vi "AR-Axis-update-parameters-GUI.vi"(8 "error in":errorcluster, 11 "Com":refnum<visa-resource-name>) -> (0 "error out":errorcluster, 1 "Axis":string[](array[string]), 2 "Connected Devices":string[](array[string]), 3 "Device Info":T4(array[cluster]) {"Microstep Size" format="%#_6f"})   [LabVIEW 2021]
uses:
  Automation/Zaber Stage/Controls/Zaber-basic-settings.ctl
  Automation/Zaber Stage/Controls/Zaber-all-settings.ctl
  <instrlib>/Zaber A Series/Public/Utility/Low Level/Convert Device Units to Position Units.vi
  <instrlib>/Zaber A Series/Public/Utility/Low Level/Convert Device Units to Speed Units.vi
  <instrlib>/Zaber A Series/Public/Utility/Low Level/Convert Device Units to Acceleration.vi
  <instrlib>/Zaber A Series/Zaber A Series.lvlib
panel:
  in  "Axis":string(combo)
  in  "All Settings":T1="cloop.duration.max"
  in  "Basic Settings":T2="comm.checksum"
  in  "Physical Units":T3(ring)
  out "To Physical Units":string
  in  "From Device":i32
  out "To Device Units":string
  in  "From Physical":dbl
  in  "Convert":enum16{"Position", "Speed", "Acceleration"}(ring)
  in  "Quit":bool
  out "Action":string
  in  "Set":bool
  in  "Get":bool
  out "Setting readback":string
  in  "Cmd parameters":string
  in  "Setting cmd":string(combo)
  in  "All/Basic(T)":bool=TRUE
  in  "Device#":string(combo)
  out "Settings":string[](array[string])
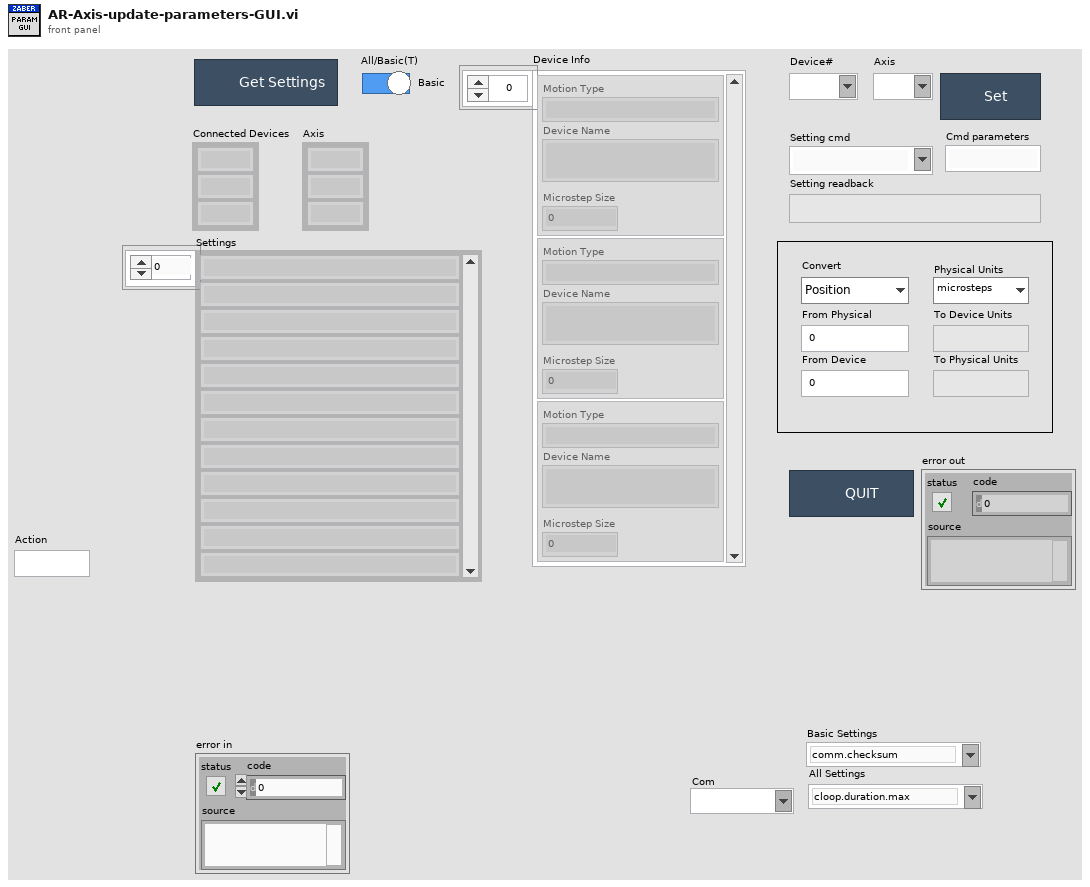
[diagram p1: front panel]
types:
  T1 = typedef "Zaber-all-settings.ctl" = string
  T2 = typedef "Zaber-basic-settings.ctl" = string
  T3 = enum16{"microsteps", "microns", "millimeters", "inches", "degrees"}
  T4 = cluster{"Motion Type":string, "Device Name":string, "Microstep Size":dbl}[]
  T5 = cluster{"Motion Type":string, "Device Name":string, "Microstep Size":dbl}
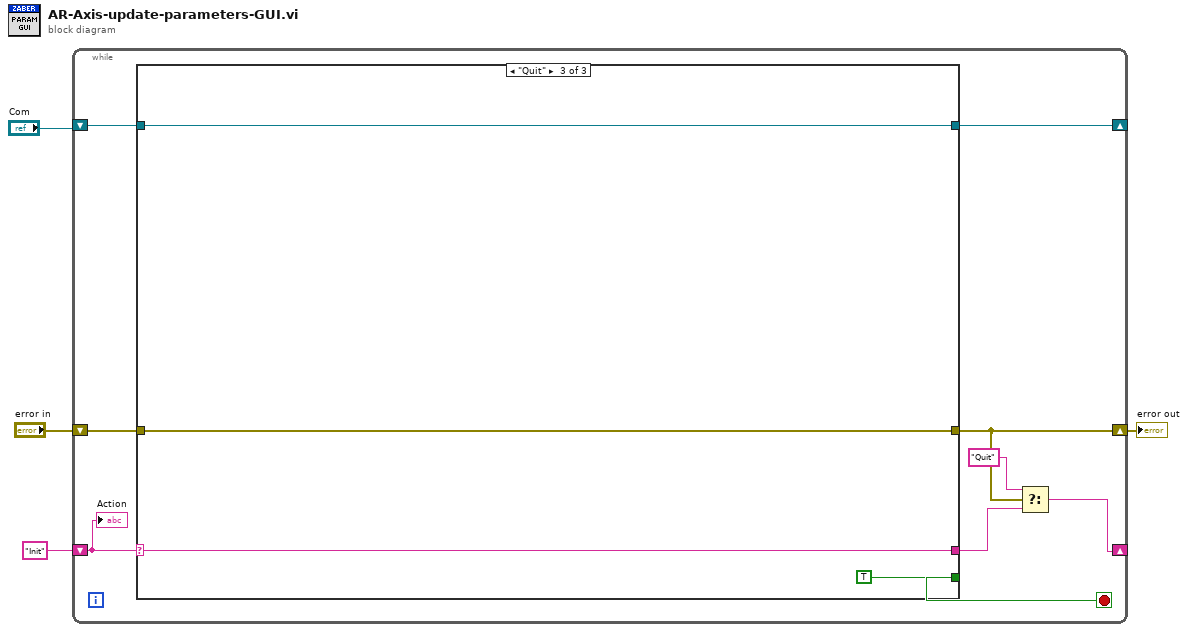
[diagram p0: block diagram]
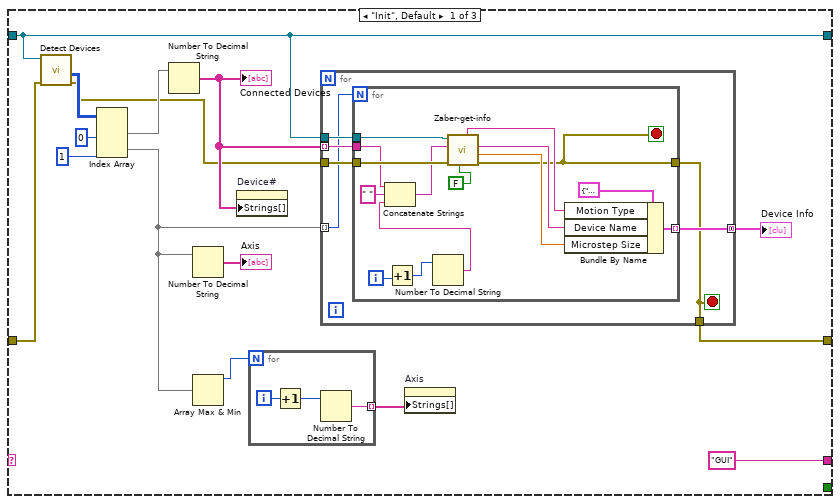
[diagram p2: hidden frame]
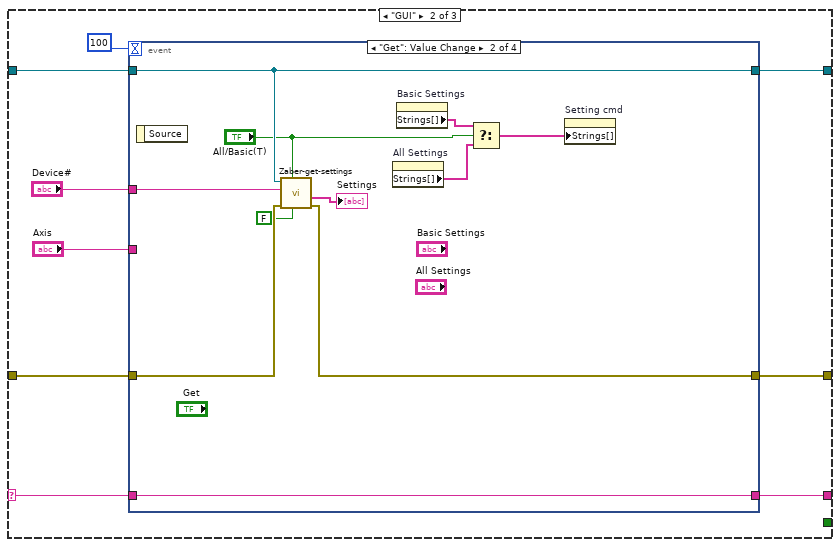
[diagram p3: hidden frame]
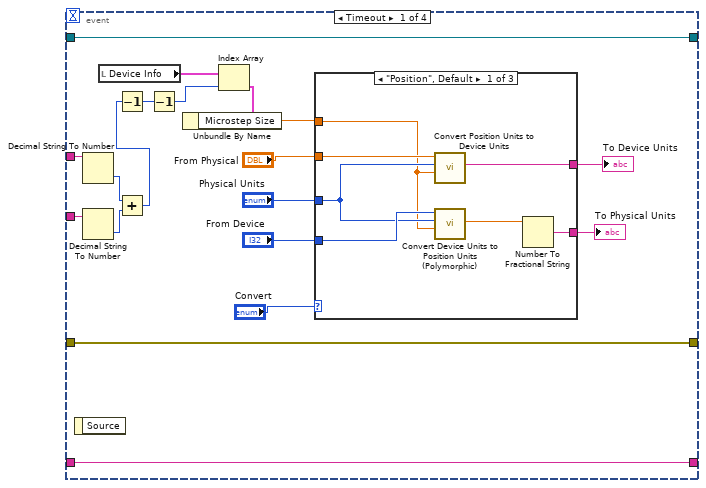
[diagram p4: hidden frame]
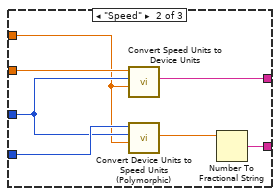
[diagram p5: hidden frame]
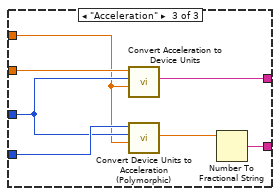
[diagram p6: hidden frame]
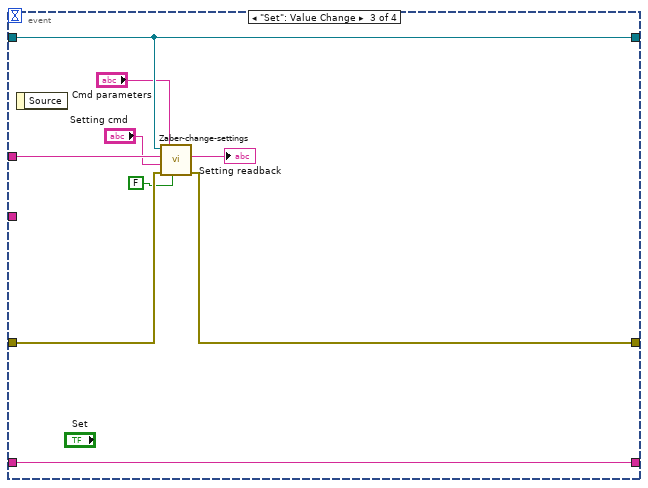
[diagram p7: hidden frame]
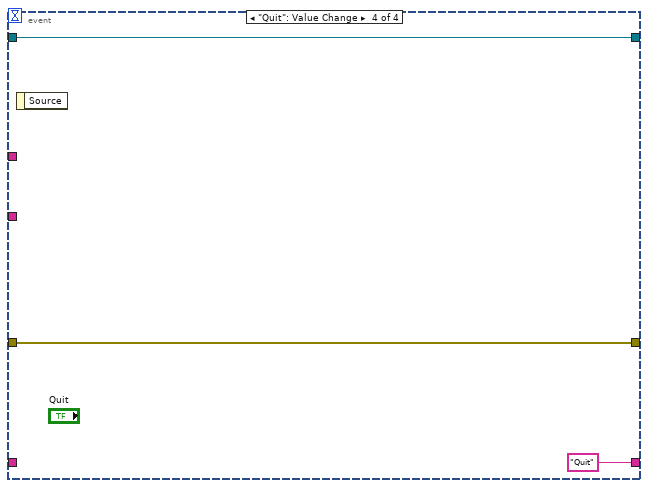
[diagram p8: hidden frame]
diagram:
  n1 = while {
    shift-right: [w12] -> _
    shift-left: "Com" -> [w10]
    shift-right: [w9] -> w3
    shift-left: "error in" -> [w11]
    shift-right: [w6] -> _
    shift-left: "Init" ("Action") -> [w13]
    stop <- w5 stop-if-true
    n2 = case shown="\"Quit\"" w13 {
      selector: w13 -> [_ w56 w126]
      tunnel: [w15 w54 w127] -> w12
      tunnel: [w27 w57 w128] -> w9
      tunnel: w11 -> [w16 w58 w128]
      tunnel: ["GUI" ("Action") w55 w126] -> w7
      tunnel: w10 -> [w15 w60 w127]
      tunnel: [_ _ TRUE] -> w5
      frame "Init", Default {
        n3 = call <instrlib>:"Detect Devices.vi"("error in (no error)"=w16, "VISA resource name"=w15) -> ("error out"=w14:errorcluster, "Axis Counts by Device"=w21:i32[][])  [unwired: 6 in, 2 out]
        n4 = Index Array(array=w21, index (col) #1=0 ("disabled index (col)"), index (col) #2=1 ("index (col)")) -> (element #1=w18:i32[], element #2=w17:i32[])  [unwired: 2 in]
        n5 = Number To Decimal String(number=w18) -> (decimal integer string=w25:string[])  [unwired: 1 in]
        "Connected Devices" <- w25
        n6 = Number To Decimal String(number=w17) -> (decimal integer string=→"Axis":string[])  [unwired: 1 in]
        n7 = Array Max & Min(array=w17) -> (max value=w23:i32)  [unwired: 3 out]
        n8 = property on="Device#" class="CmbBox"("Strings[]"=w25) -> ()  [unwired: 2 in, 2 out]
        n9 = for {
          N: w23 -> [_]
          tunnel: [w29] -> w22 mode=indexing
          i -> [w30]
          n10 = Increment(x=w30) -> (x+1=w31:i32)
          n11 = Number To Decimal String(number=w31) -> (decimal integer string=w29:string)  [unwired: 1 in]
        }
        n12 = for {
          tunnel: w25 -> [w37] mode=indexing
          tunnel: w15 -> [w36]
          tunnel: w14 -> [w35]
          tunnel: [w34] -> w28 mode=concatenating
          tunnel: [w33] -> w27
          tunnel: w17 -> [w32] mode=indexing
          stop <- w33 stop-if-true
          n13 = for {
            N: w32 -> [_]
            tunnel: w37 -> [w44]
            tunnel: w36 -> [w52]
            tunnel: [w45] -> w34 mode=indexing
            tunnel: w35 -> [w51]
            tunnel: [w43] -> w33
            i -> [w40]
            stop <- w43 stop-if-true
            n14 = Increment(x=w40) -> (x+1=w39:i32)
            n15 = Number To Decimal String(number=w39) -> (decimal integer string=w38:string)  [unwired: 1 in]
            n16 = Concatenate Strings(w44, " " ("string"), w38) -> (w41:string)
            n17 = call "Zaber-get-info.vi"("Init?"=FALSE, "error in"=w51, "Device+Axis"=w41, "Port"=w52) -> ("error out"=w43:errorcluster, "Microstep Size"=w47:dbl, "Device Name"=w49:string, "Motion Type"=w48:string)  [unwired: 3 in, 1 out]
            n18 = Bundle By Name(cluster=T5 {"Motion Type"="", "Device Name"="", "Microstep Size"=0.0} ("Cluster - Thin Border"), "Motion Type"=w48, "Device Name"=w49, "Microstep Size"=w47) -> (w45:T5)
          }
        }
        "Device Info" <- w28
        n19 = property on="Axis" class="CmbBox"("Strings[]"=w22) -> ()  [unwired: 2 in, 2 out]
      }
      frame "GUI" {
        n20 = event shown="[1] \"Get\": Value Change" {
          selector: _ -> [_ _ _ _]
          dyn-events: _ -> [_ _ _ _]
          timeout: 100 -> [_ _ _ _]
          tunnel: w60 -> [w78 w106 w117 w124]
          tunnel: "Device#" -> [w74 w112 w116 _]
          tunnel: w58 -> [w79 w111 w119 w123]
          tunnel: [w79 w108 w120 w123] -> w57
          tunnel: w56 -> [w80 w107 w121 _]
          tunnel: [w80 w107 w121 "Quit"] -> w55
          tunnel: [w78 w106 w117 w124] -> w54
          tunnel: "Axis" -> [w66 _ _ _]
          event Timeout {
            n21 = event-data() -> ()  [unwired: 1 in, 1 out]
            n22 = Decimal String To Number(string=w74) -> (number=w65:i32)  [unwired: 2 in, 1 out]
            n23 = Decimal String To Number(string=w66) -> (number=w64:i32)  [unwired: 2 in, 1 out]
            n24 = local read "Device Info"() -> (w73:T4)
            n25 = Add(x=w65, y=w64) -> (x+y=w62:i32)
            n26 = Decrement(x=w62) -> (x-1=w63:i32)
            n27 = Decrement(x=w63) -> (x-1=w72:i32)
            n28 = Index Array(array=w73, index=w72) -> (element=w71:T5)
            n29 = Unbundle By Name(w71) -> ("Microstep Size"=w70:dbl)
            n30 = case shown="\"Position\", Default" "Convert" {
              tunnel: "Physical Units" -> [w84 w91 w98]
              tunnel: "From Physical" -> [w87 w94 w101]
              tunnel: w70 -> [w83 w90 w97]
              tunnel: [w86 w93 w100] -> w69
              tunnel: "From Device" -> [w85 w92 w99]
              tunnel: [w81 w88 w95] -> w67
              frame "Position", Default {
                n31 = call <instrlib>:"Convert Position Units to Device Units.vi"("Microstep Size (0)"=w83, "Units (0: microsteps)"=w84, "Position (0)"=w87) -> ("Device Position (String)"=w86:string)  [unwired: 6 in, 2 out]
                n32 = call-poly <instrlib>:"Convert Device Units to Position Units (Polymorphic).vi"("Microstep Size (0)"=w83, "Units (0: microsteps)"=w84, "Device Position (0)"=w85) -> ("Position"=w82:dbl)  [unwired: 8 in]
                n33 = Number To Fractional String(number=w82) -> (F-format string=w81:string)  [unwired: 3 in]
              }
              frame "Speed" {
                n34 = call <instrlib>:"Convert Speed Units to Device Units.vi"("Microstep Size (0)"=w90, "Units (0: device speed units)"=w91, "Speed (0)"=w94) -> ("Device Speed (String)"=w93:string)  [unwired: 6 in, 2 out]
                n35 = call-poly <instrlib>:"Convert Device Units to Speed Units (Polymorphic).vi"("Microstep Size (0)"=w90, "Units (0: device speed units)"=w91, "Device Speed (0)"=w92) -> ("Speed"=w89:dbl)  [unwired: 8 in]
                n36 = Number To Fractional String(number=w89) -> (F-format string=w88:string)  [unwired: 3 in]
              }
              frame "Acceleration" {
                n37 = call <instrlib>:"Convert Acceleration to Device Units.vi"("Microstep Size (0)"=w97, "Units (0: device acceleration units)"=w98, "Acceleration (0)"=w101) -> ("Device Acceleration (String)"=w100:string)  [unwired: 6 in, 2 out]
                n38 = call-poly <instrlib>:"Convert Device Units to Acceleration (Polymorphic).vi"("Microstep Size (0)"=w97, "Units (0: device acceleration units)"=w98, "Device Acceleration (0)"=w99) -> ("Acceleration"=w96:dbl)  [unwired: 8 in]
                n39 = Number To Fractional String(number=w96) -> (F-format string=w95:string)  [unwired: 3 in]
              }
            }
            "To Device Units" <- w69
            "To Physical Units" <- w67
          }
          event "Get": Value Change {
            n40 = event-data() -> ()  [unwired: 1 in, 1 out]
            n41 = call "Zaber-get-settings.vi"("Init?"=FALSE, "All/Basic(T)"="All/Basic(T)", "error in"=w111, "Device#"=w112, "Com"=w106) -> ("error out"=w108:errorcluster, "Settings"=→"Settings":string[])  [unwired: 1 in, 4 out]
            n42 = property on="All Settings" class="CmbBox (strict)"() -> ("Strings[]"=w104:string[])  [unwired: 2 in, 2 out]
            n43 = property on="Basic Settings" class="CmbBox (strict)"() -> ("Strings[]"=w103:string[])  [unwired: 2 in, 2 out]
            n44 = Select(t=w103, s="All/Basic(T)", f=w104) -> (s? t:f=w102:string[])
            n45 = property on="Setting cmd" class="CmbBox"("Strings[]"=w102) -> ()  [unwired: 2 in, 2 out]
          }
          event "Set": Value Change {
            n46 = event-data() -> ()  [unwired: 1 in, 1 out]
            n47 = call "Zaber-change-settings.vi"("Init?"=FALSE, "Cmd parameters"="Cmd parameters", "error in"=w119, "Setting cmd"="Setting cmd", "Device#"=w116, "Com"=w117) -> ("error out"=w120:errorcluster, "Setting readback"=→"Setting readback":string)  [unwired: 3 in, 1 out]
          }
          event "Quit": Value Change {
            n48 = event-data() -> ()  [unwired: 1 in, 1 out]
          }
        }
      }
      frame "Quit" {
      }
    }
    n49 = Select(t="Quit" ("Action"), s=w9, f=w7) -> (s? t:f=w6:string)
    "Action" <- w13
  }
  "error out" <- w3
